vi "GetProperties.vi"(8 "error in":errorcluster, 11 "Numeric Text in":refnum<class "Digital.lvclass">) -> (0 "error out":errorcluster, 3 "Numeric Text out":refnum<class "Digital.lvclass">)   [LabVIEW 2014, in "Raspberry Pi Compatible Compiler for LabVIEW.lvlib" / "Digital.lvclass"]
uses:
  Digital.lvclass
  Digital.lvclass/Digital.ctl
  Numeric/Numeric.lvclass
  NumericText/NumericText.lvclass
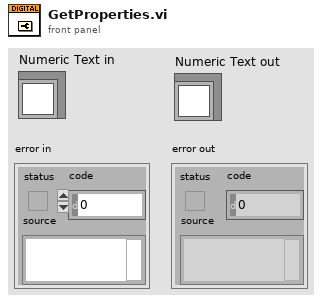
[diagram p1: front panel]
types:
  T1 = typedef "LVFormatAndPrecisionTypeDef.ctl" = cluster{"Format":u8, "Precision":u8}
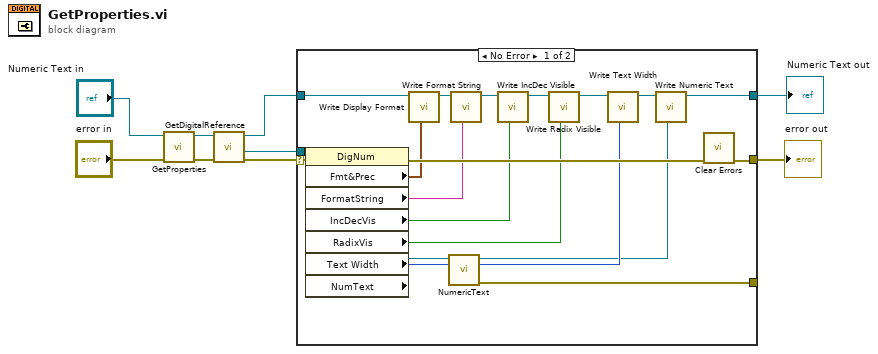
[diagram p0: block diagram]
diagram:
  n1 = call-parent "GetProperties.vi"("error in"="error in", "Numeric in"="Numeric Text in") -> ("error out"=w3:errorcluster, "Numeric out"=w4:refnum<class "Digital.lvclass">)  [unwired: 8 in]
  n2 = call "GetDigitalReference.vi"("error in"=w3, "Numeric Text in"=w4) -> ("error out"=w8:errorcluster, "Digital reference"=w7:refnum<vi>, "Numeric Text out"=w6:refnum<class "Digital.lvclass">)  [unwired: 7 in]
  n3 = case shown="No Error" w8 {
    selector: w8 -> [w28 w30]
    tunnel: [w11 w30] -> w9
    tunnel: w7 -> [w27 _]
    tunnel: w6 -> [w24 w29]
    tunnel: [w13 w29] -> w5
    tunnel: [w10 _] -> _
    frame No Error {
      n4 = property class="DigNum"(reference=w27, error in=w28) -> (error out=w26:errorcluster, "Fmt&Prec"=w25:T1, "FormatString"=w22:string, "IncDecVis"=w20:bool, "RadixVis"=w18:bool, "Text Width"=w16:u32, "NumText"=w15:refnum<vi>)  [unwired: 1 out]
      n5 = call "Write Display Format.vi"("Display Format"=w25, "NumericText in"=w24) -> ("NumericText out"=w23:refnum<class "Digital.lvclass">)  [unwired: 7 in]
      n6 = call "NumericText.vi"("GObj Refnum"=w15) -> ("error out"=w10:errorcluster, "Numeric Text out"=w12:refnum<class "NumericText.lvclass">)  [unwired: 9 in]
      n7 = call "Write Format String.vi"("Format String"=w22, "NumericText in"=w23) -> ("NumericText out"=w21:refnum<class "Digital.lvclass">)  [unwired: 7 in]
      n8 = call "Write IncDec Visible.vi"("IncDec Visible"=w20, "Digital in"=w21) -> ("Digital out"=w19:refnum<class "Digital.lvclass">)  [unwired: 7 in]
      n9 = call "Write Radix Visible.vi"("Radix Visible"=w18, "Digital in"=w19) -> ("Digital out"=w17:refnum<class "Digital.lvclass">)  [unwired: 7 in]
      n10 = call "Write Text Width.vi"("Text Width"=w16, "Digital in"=w17) -> ("Digital out"=w14:refnum<class "Digital.lvclass">)  [unwired: 7 in]
      n11 = call "Write Numeric Text.vi"("NumericText"=w12, "Digital in"=w14) -> ("Digital out"=w13:refnum<class "Digital.lvclass">)  [unwired: 7 in]
      n12 = call <vilib>:"Clear Errors.vi"("error in (no error)"=w26) -> ("error out"=w11:errorcluster)  [unwired: 5 in, 1 out]
    }
    frame Error {
    }
  }
  "error out" <- w9
  "Numeric Text out" <- w5
